vi "GE5565 DMA Read Interrupt (U64) Cluster 2.vi"(6 "timeout (1000 ms)":u32=1000, 8 "error in (no error)":errorcluster, 10 "offset (0)":u32, 11 "VMIC reference in":T1) -> (0 "error out":errorcluster, 2 "buffer":u64[](array[numeric]), 3 "VMIC reference out":T1)   [LabVIEW 2016]
uses:
  <vilib>/Instr/_visa.llb/Select Event Type.ctl
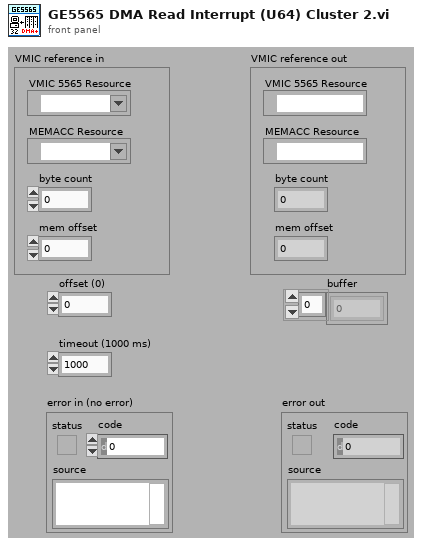
[diagram p1: front panel]
types:
  T1 = cluster{"VMIC 5565 Resource":refnum<visa-resource-name>, "MEMACC Resource":refnum<visa-resource-name>, "byte count":u32, "mem offset":u32}
  T2 = typedef "Select Event Type.ctl" = u32
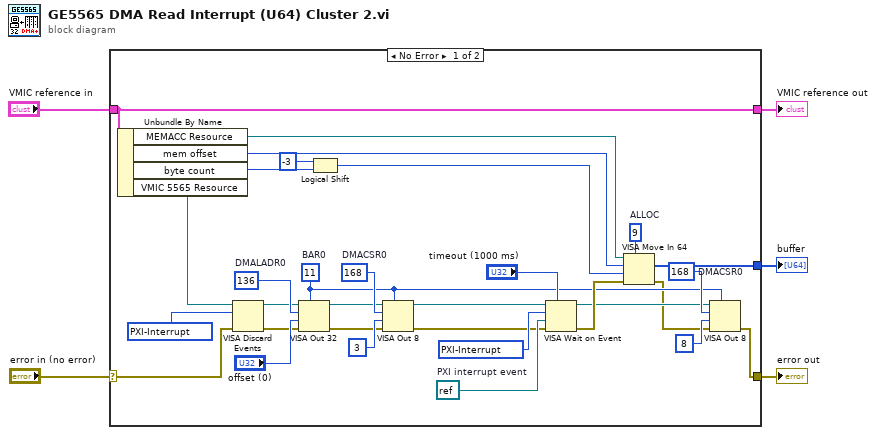
[diagram p0: block diagram]
diagram:
  n1 = case shown="No Error" "error in (no error)" {
    selector: "error in (no error)" -> [w24 w37]
    tunnel: "VMIC reference in" -> [w18 w38]
    tunnel: [w18 w38] -> w2
    tunnel: [w9 w37] -> w4
    tunnel: [w29 _] -> w1
    frame No Error {
      w30 = u16 9  # ALLOC
      w11 = u16 11  # BAR0
      w26 = refnum<visa-resource-name> refnum  # PXI interrupt event
      w14 = u32 168  # DMACSR0
      w21 = T2 1073684514 items=["ServiceRequest"=1073684491, "Trigger"=3221168138, "Clear"=1073684493, "VXI-Signal"=1073684512, "VXI/VME-Interrupt"=3221168161, "VXI/VME-Sysfail"=1073684509, "VXI/VME-Sysreset"=1073684510, "GPIB-CIC"=1073684498, "GPIB-Talk"=1073684499, "GPIB-Listen"=1073684500, "PXI-Interrupt"=1073684514, "AllEnabled"=1073709055] ("Event Type")
      w27 = T2 1073684514 items=["ServiceRequest"=1073684491, "Trigger"=3221168138, "Clear"=1073684493, "VXI-Signal"=1073684512, "VXI/VME-Interrupt"=3221168161, "VXI/VME-Sysfail"=1073684509, "VXI/VME-Sysreset"=1073684510, "GPIB-CIC"=1073684498, "GPIB-Talk"=1073684499, "GPIB-Listen"=1073684500, "PXI-Interrupt"=1073684514, "AllEnabled"=1073709055] ("Event Type")
      w35 = u32 168  # DMACSR0
      w36 = u32 136  # DMALADR0
      n2 = Unbundle By Name(w18) -> ("MEMACC Resource"=w16:refnum<visa-resource-name>, "mem offset"=w17:u32, "byte count"=w8:u32, "VMIC 5565 Resource"=w19:refnum<visa-resource-name>)
      n3 = VISA Discard Events(8:w24, 10:w21, 11:w19) -> (0:w22:errorcluster, 3:w23:refnum<visa-resource-name>)  [unwired: 1 in]
      n4 = VISA Out 32(7:w11, 8:w22, 9:"offset (0)", 10:w36, 11:w23) -> (0:w32:errorcluster, 3:w33:refnum<visa-resource-name>)
      n5 = Logical Shift(y=i16 -3, x=w8) -> (x << y=w7:u32)
      n6 = VISA Out 8(7:w11, 8:w32, 9:u8 3 ("value (0)"), 10:w35, 11:w33) -> (0:w15:errorcluster, 3:w25:refnum<visa-resource-name>)
      n7 = VISA Wait on Event(7:"timeout (1000 ms)", 8:w15, 9:w26, 10:w27, 11:w25) -> (0:w20:errorcluster, 3:w12:refnum<visa-resource-name>)  [unwired: 2 out]
      n8 = VISA Move In 64(7:w30, 8:w20, 9:w7, 10:w17, 11:w16) -> (0:w10:errorcluster, 2:w29:u64[])  [unwired: 1 out]
      n9 = VISA Out 8(7:w11, 8:w10, 9:u8 8 ("value (0)"), 10:w14, 11:w12) -> (0:w9:errorcluster)  [unwired: 1 out]
    }
    frame Error {
    }
  }
  "error out" <- w4
  "VMIC reference out" <- w2
  "buffer" <- w1
